vi "Write Source PDF File [ ] test.vi"(0 "PDF Report IN":refnum<class "PDF Report Class.lvclass">=refnum, 11 "error in (no error)":errorcluster) -> (4 "PDF Report OUT":refnum<class "PDF Report Class.lvclass">, 15 "error out":errorcluster)   [LabVIEW 2020, in "Exaprom PDF.lvlib"]
doc: "Version 2.0\nDeveloped by Jean-Marc Simard\nCopyright © 2012, Exaprom Inc.\nAll rights reserved.\nLicense: BSD\n\nWith iTextSharp 4.1.6 (http://itextsharp.sourceforge.net)\nunder Mozilla Public License Version 1.1\n(http://www.mozilla.org/MPL/MPL-1.1.html)"
uses:
  <userlib>/labview-PDF-writer-master/Exaprom PDF.lvlib
  <userlib>/labview-PDF-writer-master/LV Class/PDF Report Class/PDF Report Class.lvclass
  <userlib>/labview-PDF-writer-master/LV Class/Fonts Class/Font Class.lvclass
  <userlib>/labview-PDF-writer-master/LV Class/Header and Footer Class/Header and Footer Class.lvclass
  <userlib>/labview-PDF-writer-master/Controls/Concatenate Controls/PDF File and position.ctl
  <userlib>/labview-PDF-writer-master/Controls/Concatenate Controls/PDF file source.ctl
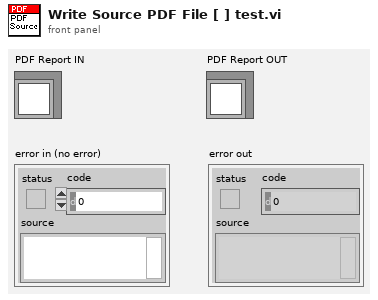
[diagram p1: front panel]
types:
  T1 = typedef "Exaprom PDF.lvlib/PDF File and position.ctl" = cluster{"Path":path, "Pages":string, "Source":T2, "Start at page old":i32, "Start at page new":i32, "Owner password":string}
  T2 = typedef "Exaprom PDF.lvlib/PDF file source.ctl" = enum16{"PDF Report", "File to add"}
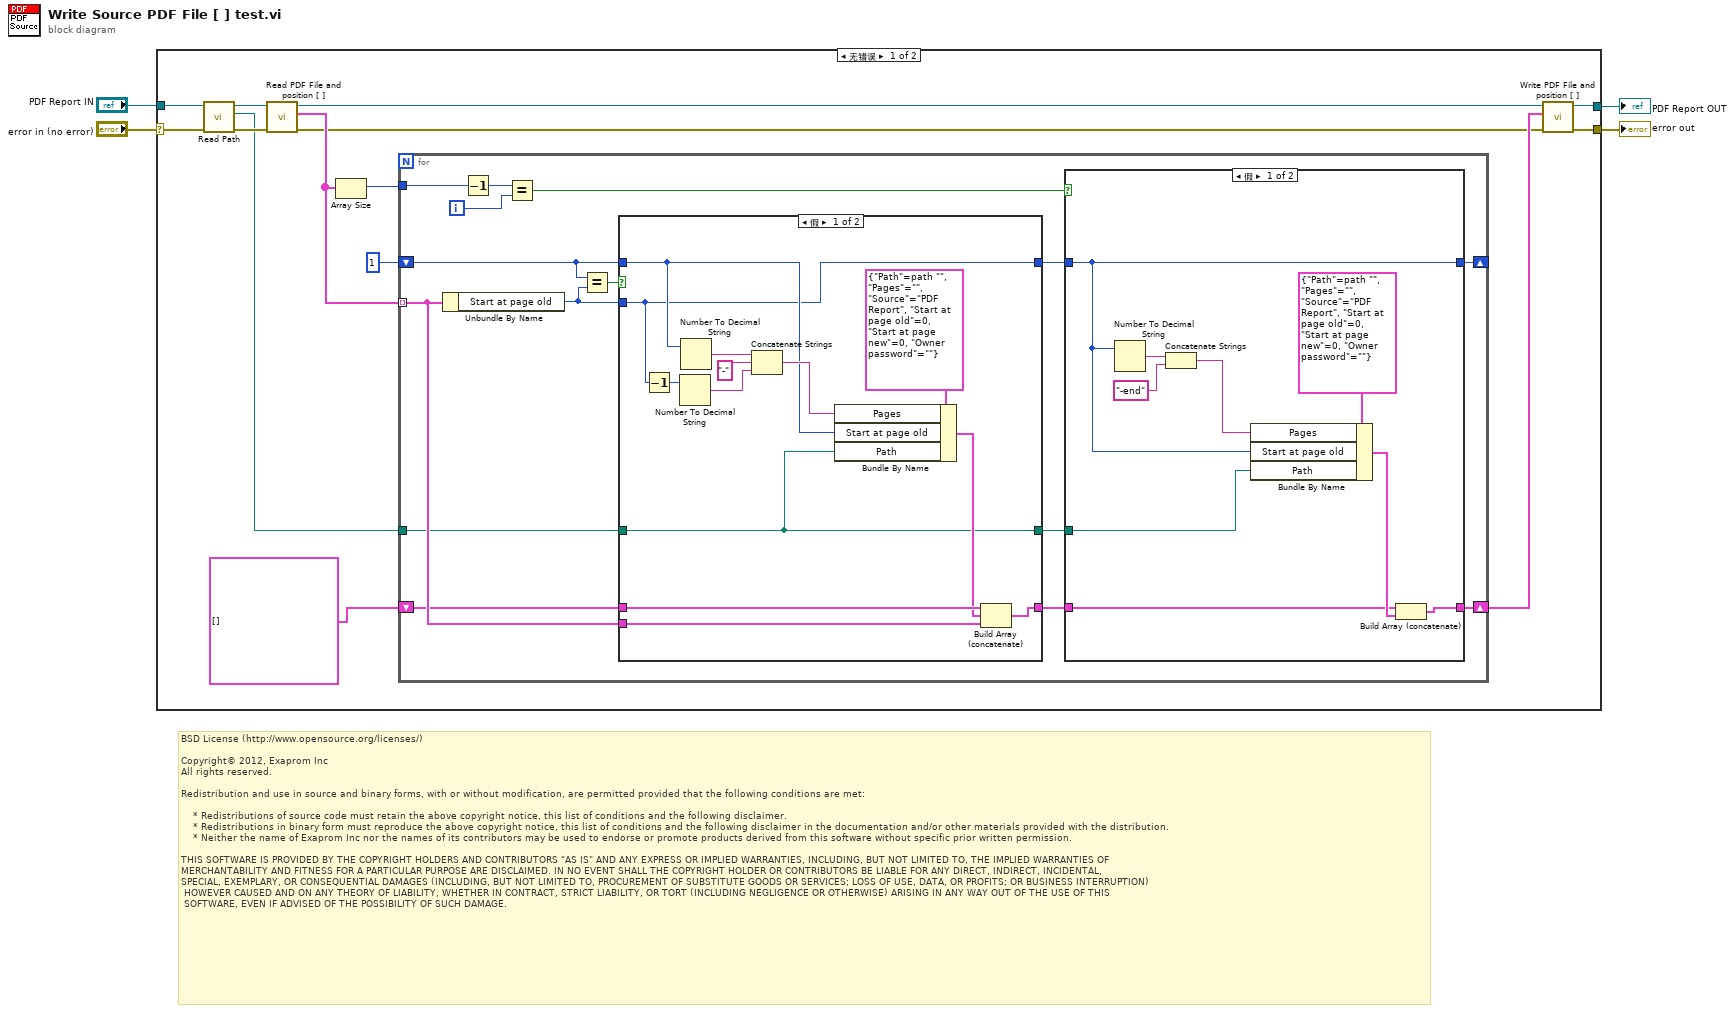
[diagram p0: block diagram]
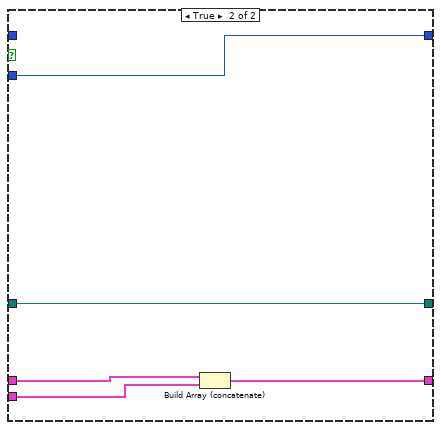
[diagram p3: hidden frame]
diagram:
  # "BSD License (http://www.opensource.org/licenses/)\n\nCopyright© 2012, Exaprom Inc\nAll rights reserved.\n\nRedistribution and use in source and binary forms, with or without modification, are permitted provided that the following conditions are met:\n\n    * Redistributions of source code must retain the above copyright notice, this list of conditions and the following disclaimer.\n    * Redistributions in binary form must reproduce the above copyright notice, this list of conditions and the following disclaimer in the documentation and/or other materials provided with the distribution.\n    * Neither the name of Exaprom Inc nor the names of its contributors may be used to endorse or promote products derived from this software without specific prior written permission.\n\nTHIS SOFTWARE IS PROVIDED BY THE COPYRIGHT HOLDERS AND CONTRIBUTORS \"AS IS\" AND ANY EXPRESS OR IMPLIED WARRANTIES, INCLUDING, BUT NOT LIMITED TO, THE IMPLIED WARRANTIES OF \nMERCHANTABILITY AND FITNESS FOR A PARTICULAR PURPOSE ARE DISCLAIMED. IN NO EVENT SHALL THE COPYRIGHT HOLDER OR CONTRIBUTORS BE LIABLE FOR ANY DIRECT, INDIRECT, INCIDENTAL,\nSPECIAL, EXEMPLARY, OR CONSEQUENTIAL DAMAGES (INCLUDING, BUT NOT LIMITED TO, PROCUREMENT OF SUBSTITUTE GOODS OR SERVICES; LOSS OF USE, DATA, OR PROFITS; OR BUSINESS INTERRUPTION)\n HOWEVER CAUSED AND ON ANY THEORY OF LIABILITY, WHETHER IN CONTRACT, STRICT LIABILITY, OR TORT (INCLUDING NEGLIGENCE OR OTHERWISE) ARISING IN ANY WAY OUT OF THE USE OF THIS\n SOFTWARE, EVEN IF ADVISED OF THE POSSIBILITY OF SUCH DAMAGE."
  n1 = case shown="无错误" "error in (no error)" {
    selector: "error in (no error)" -> [w15 w64]
    tunnel: "PDF Report IN" -> [w5 w63]
    tunnel: [w12 w63] -> w3
    tunnel: [w13 w64] -> w2
    frame No Error {
      n2 = call-dynamic "Read Path.vi"("error in (no error)"=w15, "PDF Report Class in"=w5) -> ("error out"=w8:errorcluster, "Path"=w7:path, "PDF Report Class out"=w6:refnum<class "PDF Report Class.lvclass">)  [unwired: 7 in]
      n3 = call-dynamic "Read PDF File and position [ ].vi"("error in (no error)"=w8, "PDF Report Class in"=w6) -> ("error out"=w10:errorcluster, "PDF File and position [ ]"=w14:T1[], "PDF Report Class out"=w9:refnum<class "PDF Report Class.lvclass">)  [unwired: 7 in]
      n4 = Array Size(array=w14) -> (size(s)=w16:i32)
      n5 = for {
        tunnel: w14 -> [w33] mode=indexing
        shift-right: [w24] -> _
        shift-left: 1 ("Start at page") -> [w22]
        shift-right: [w26] -> w11
        shift-left: T1[] [] -> [w31]
        tunnel: w16 -> [w30]
        tunnel: w7 -> [w20]
        i -> [w29]
        n6 = Unbundle By Name(w33) -> ("Start at page old"=w21:i32)
        n7 = Decrement(x=w30) -> (x-1=w28:i32)
        n8 = Equal?(x=w28, y=w29) -> (x = y?=w27:bool)
        n9 = Equal?(x=w22, y=w21) -> (x = y?=w32:bool)
        n10 = case shown="假" w32 {
          tunnel: [w46 w60] -> w23
          tunnel: w22 -> [w49 _]
          tunnel: w33 -> [w52 w61]
          tunnel: [w51 w62] -> w25
          tunnel: w31 -> [w53 w59]
          tunnel: w21 -> [w46 w60]
          tunnel: w20 -> [w45 w58]
          tunnel: [w45 w58] -> w19
          frame False {
            n11 = Decrement(x=w46) -> (x-1=w50:i32)
            n12 = Number To Decimal String(number=w50) -> (decimal integer string=w56:string)  [unwired: 1 in]
            n13 = Number To Decimal String(number=w49) -> (decimal integer string=w57:string)  [unwired: 1 in]
            n14 = Concatenate Strings(w57, "-" ("string"), w56) -> (w54:string)
            n15 = Bundle By Name(cluster=T1 {"Path"=path "", "Pages"="", "Source"=enum."PDF Report", "Start at page old"=0, "Start at page new"=0, "Owner password"=""} ("PDF File and position"), "Pages"=w54, "Start at page old"=w49, "Path"=w45) -> (w47:T1)
            n16 = Build Array (concatenate)(w53, w47, w52) -> (w51:T1[])
          }
          frame True {
            n17 = Build Array (concatenate)(w59, w61) -> (w62:T1[])
          }
        }
        n18 = case shown="假" w27 {
          tunnel: [w35 w44] -> w26
          tunnel: w25 -> [w36 w44]
          tunnel: [w38 w43] -> w24
          tunnel: w23 -> [w38 w43]
          tunnel: w19 -> [w34 _]
          frame False {
            n19 = Number To Decimal String(number=w38) -> (decimal integer string=w42:string)  [unwired: 1 in]
            n20 = Concatenate Strings(w42, "-end" ("string")) -> (w40:string)
            n21 = Bundle By Name(cluster=T1 {"Path"=path "", "Pages"="", "Source"=enum."PDF Report", "Start at page old"=0, "Start at page new"=0, "Owner password"=""} ("PDF File and position"), "Pages"=w40, "Start at page old"=w38, "Path"=w34) -> (w37:T1)
            n22 = Build Array (concatenate)(w36, w37) -> (w35:T1[])
          }
          frame True {
          }
        }
      }
      n23 = call-dynamic "Write PDF File and position [ ].vi"("error in (no error)"=w10, "PDF File and position [ ]"=w11, "PDF Report Class in"=w9) -> ("error out"=w13:errorcluster, "PDF Report Class out"=w12:refnum<class "PDF Report Class.lvclass">)  [unwired: 7 in]
    }
    frame Error {
    }
  }
  "PDF Report OUT" <- w3
  "error out" <- w2
